vi "Load Config.vi"(6 "Constants":refnum<class "Sequence Constants.lvclass">, 8 "error in (no error)":refnum<class "MultiErrors.lvclass">, 10 "Config Element":refnum<class "Config Element.lvclass">, 11 "OutOfRange Condition Config in":refnum<class "OutOfRange Condition Config.lvclass">) -> (0 "error out":refnum<class "MultiErrors.lvclass">, 3 "OutOfRange Condition Config out":refnum<class "OutOfRange Condition Config.lvclass">)   [LabVIEW 2020, in "VolatusSeqConfig.lvlib" / "OutOfRange Condition Config.lvclass"]
uses:
  OutOfRange Condition Config.lvclass
  VolatusErrorUtilities/MultiErrors/MultiErrors.lvclass
  lv-cdm/CDM-Config/Config Element/Config Element.lvclass
  OutOfRange Condition Config.lvclass/OutOfRange Condition Config.ctl
  Sequence Constants/Sequence Constants.lvclass
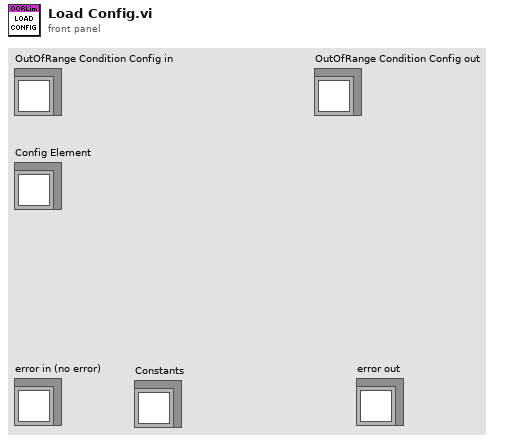
[diagram p1: front panel]
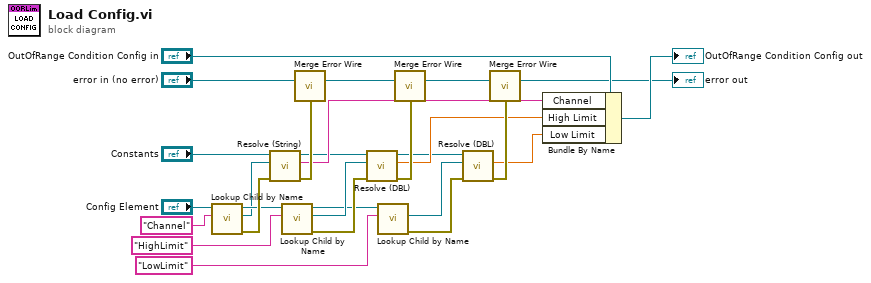
[diagram p0: block diagram]
diagram:
  n1 = call "Lookup Child by Name.vi"("Name"="Channel", "Config Element in"="Config Element") -> ("error out"=w27:errorcluster, "Child"=w17:refnum<class "Config Element.lvclass">, "Config Element out"=w18:refnum<class "Config Element.lvclass">)  [unwired: 6 in, 1 out]
  n2 = call "Resolve (String).vi"("error in (no error)"=w27, "Element"=w17, "Sequence Constants in"="Constants") -> ("error out"=w24:errorcluster, "String Value"=w10:string, "Sequence Constants out"=w2:refnum<class "Sequence Constants.lvclass">)  [unwired: 6 in]
  n3 = call "Lookup Child by Name.vi"("Name"="HighLimit", "Config Element in"=w18) -> ("error out"=w26:errorcluster, "Child"=w16:refnum<class "Config Element.lvclass">, "Config Element out"=w14:refnum<class "Config Element.lvclass">)  [unwired: 6 in, 1 out]
  n4 = call "Merge Error Wire.vi"("error in (no error)"=w24, "MultiErrors in"="error in (no error)") -> ("MultiErrors out"=w6:refnum<class "MultiErrors.lvclass">)  [unwired: 13 in]
  n5 = call "Resolve (DBL).vi"("error in (no error)"=w26, "Element"=w16, "Sequence Constants in"=w2) -> ("error out"=w23:errorcluster, "DBL Value"=w9:dbl, "Sequence Constants out"=w3:refnum<class "Sequence Constants.lvclass">)  [unwired: 6 in]
  n6 = call "Lookup Child by Name.vi"("Name"="LowLimit", "Config Element in"=w14) -> ("error out"=w25:errorcluster, "Child"=w15:refnum<class "Config Element.lvclass">)  [unwired: 6 in, 2 out]
  n7 = call "Merge Error Wire.vi"("error in (no error)"=w23, "MultiErrors in"=w6) -> ("MultiErrors out"=w5:refnum<class "MultiErrors.lvclass">)  [unwired: 13 in]
  n8 = call "Resolve (DBL).vi"("error in (no error)"=w25, "Element"=w15, "Sequence Constants in"=w3) -> ("error out"=w22:errorcluster, "DBL Value"=w8:dbl)  [unwired: 6 in, 1 out]
  n9 = call "Merge Error Wire.vi"("error in (no error)"=w22, "MultiErrors in"=w5) -> ("MultiErrors out"=→"error out":refnum<class "MultiErrors.lvclass">)  [unwired: 13 in]
  n10 = Bundle By Name(cluster="OutOfRange Condition Config in", "Channel"=w10, "High Limit"=w9, "Low Limit"=w8) -> (→"OutOfRange Condition Config out":refnum<class "OutOfRange Condition Config.lvclass">)
